vi "Bool_send.vi"(8 "连接ID":refnum<k5>, 10 "msg.data":bool, 11 "topic":string="/chatter") -> (0 "连接ID输出":refnum<k5>)   [LabVIEW 2014]
panel:
  out "JSON":string
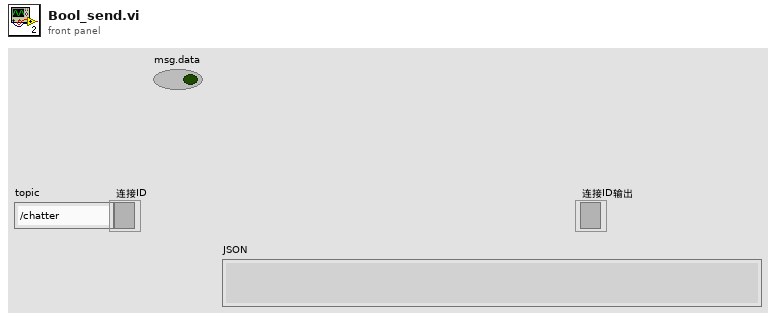
[diagram p1: front panel]
types:
  T1 = cluster{"op":string, "topic":string, "msg":cluster{"data":bool}}
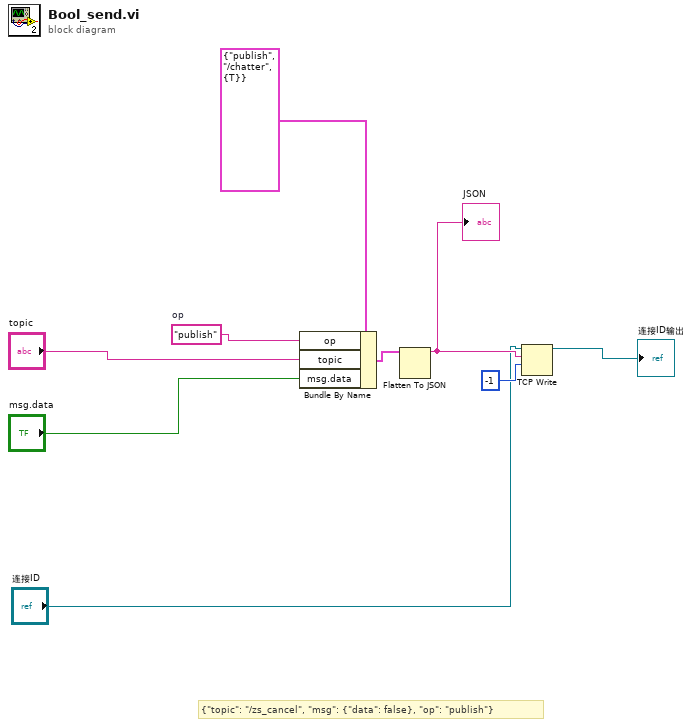
[diagram p0: block diagram]
diagram:
  w8 = "publish"  # op
  # "{\"topic\": \"/zs_cancel\", \"msg\": {\"data\": false}, \"op\": \"publish\"}"
  n1 = Bundle By Name(cluster=T1 {"op"="publish", "topic"="/chatter", "msg"={"data"=TRUE}}, "op"=w8, "topic"="topic", "msg.data"="msg.data") -> (w6:T1)
  n2 = Flatten To JSON(anything=w6) -> (JSON string=w4:string)  [unwired: 2 in, 1 out]
  "JSON" <- w4
  n3 = TCP Write(connection ID="连接ID", data in=w4, 9:-1 ("超时毫秒(25000)")) -> (connection ID out=→"连接ID输出":refnum<k5>)  [unwired: 1 in, 2 out]
